vi "GMLAN Diagnostics Engine.vi"(8 "error in (no error)":errorcluster, 11 "State Variables":T1={"TCP Refs"={"Connection List"=refnum, "listener ID"=refnum}, "Stop"=refnum, "Top VI"=refnum, "Parameters"={"Name"="", "PID Lookup"=variant, "DID Lookup"=variant, "Section Properties"={"CAN"={"Database File"=path "", "CAN Interface"=enum."CAN0", "Baud Rate"=0, "Diagnostic Protocol"=enum."GMLAN", "Transport Protocol"=enum."ISO TP - Normal Mode", "Transmit ID"=0, "Receive ID"=0, "Transmit Extension"=0, "Receive Extension"=0, "Receive UUDT ID"=0, "Enable Stream"=TRUE, "VW TP Channel ID"=0}, "DPIDs"=[], "DTC descriptor"={"DTC Byte Length"=2, "Status Byte Length"=1, "Add Data Byte Length"=1, "Byte Order"=enum."Motorola"}, "PIDs"=[], "DIDs"=[], "CPIDs"=[]}, "ChanRefs"={"ToVS.PIDs"={"Name"="", "Write to VS Engine FIFO"=refnum, "Pairs"={"Refs"=[], "Values"=[]}}, "ToVS.DIDs"={"Name"="", "Write to VS Engine FIFO"=refnum, "Pairs"={"Refs"=[], "Values"=[]}}, "ToVS.DTCs"={"Name"="", "Write to VS Engine FIFO"=refnum, "Pairs"={"Refs"=[], "Values"=[]}}, "ToVS.DTCCount"={"Name"="", "Write to VS Engine FIFO"=refnum, "Pairs"={"Refs"=[], "Values"=[]}}, "ToVS.Success"={"Name"="", "Write to VS Engine FIFO"=refnum, "Pairs"={"Refs"=[], "Values"=[]}}, "FromVS.CPIDs"={"Name"="", "Read from VS Engine FIFO"=refnum, "Pairs"={"Refs"=[], "Values"=[]}}, "Cmds"={"Name"="", "Write to VS Engine FIFO"=refnum, "Read from VS Engine FIFO"=refnum, "Pairs"={"Chan Refs"=[], "Prev. Values"=[]}}}, "CPID Lookup"=variant, "DPID Lookup"=variant}, "ADCS Connection"={"Diag CAN Handle"=0, "Transport Protocol"=enum."ISO TP - Normal Mode", "Receive Address Extension"=0, "Transmit Address Extension"=0, "Receive CAN Id"=0, "Transmit CAN Id"=0, "Diag CAN Queue"=refnum, "Log Frames ?"=FALSE, "My TP Address"=0, "Other TP Address"=0, "T1"=0, "T2"=0, "T3"=0, "T4"=0, "Tx SN"=0, "Block Size"=0, "Rx SN"=0, "VW TP Initialized?"=FALSE, "Tx block no"=0, "baud rate"=0, "Interface"="", "Channel Diag CAN Handle"=0, "UDP Connection ID"=refnum, "TCP Connection ID"=refnum, "Target IP Addr"=0, "Source Address"=0, "Target Address"=0, "Send Header NACK?"=FALSE, "DLL Handle"=0, "NAD"=0, "Time Stamp read first"=0.0, "Time Stamp read last"=0.0, "Time Stamp write first"=0.0, "Time Stamp write last"=0.0, "Time Stamp write"=0.0, "Time Stamp read"=0.0}, "XNET References"={"Database"="", "GMLAN DPID Session"="", "Cluster"=""}, "BufferedCmds"=refnum, "XNETEngine (GMLAN)"=refnum} {"Parameters"."ChanRefs"."Cmds"."Pairs"."Chan Refs" format="%.0x"; "Parameters"."ChanRefs"."ToVS.Success"."Pairs"."Refs" format="%.0x"; "Parameters"."ChanRefs"."ToVS.DTCCount"."Pairs"."Refs" format="%.0x"; "Parameters"."ChanRefs"."ToVS.DTCs"."Pairs"."Refs" format="%.0x"; "Parameters"."ChanRefs"."ToVS.PIDs"."Pairs"."Refs" format="%.0x"; "Parameters"."ChanRefs"."ToVS.DIDs"."Pairs"."Refs" format="%.0x"; "Parameters"."Section Properties"."CPIDs"."Signals"."Byte Order" items=["Little Endian", "Big Endian"]; "Parameters"."Section Properties"."CPIDs"."Signals"."Data Type" items=["Signed", "Unsigned", "IEEE Float"]; "Parameters"."Section Properties"."DIDs"."Signals"."Byte Order" items=["Little Endian", "Big Endian"]; "Parameters"."Section Properties"."DIDs"."Signals"."Data Type" items=["Signed", "Unsigned", "IEEE Float"]; "Parameters"."Section Properties"."CAN"."VW TP Channel ID" format="%.0x"; "Parameters"."Section Properties"."CAN"."Receive UUDT ID" format="%.0x"; "Parameters"."Section Properties"."CAN"."Receive Extension" format="%.0x"; "Parameters"."Section Properties"."CAN"."Transmit Extension" format="%.0x"; "Parameters"."Section Properties"."CAN"."Receive ID" format="%.0x"; "Parameters"."Section Properties"."CAN"."Transmit ID" format="%.0x"; "Parameters"."Section Properties"."PIDs"."Signals"."Byte Order" items=["Little Endian", "Big Endian"]; "Parameters"."Section Properties"."PIDs"."Signals"."Data Type" items=["Signed", "Unsigned", "IEEE Float"]}) -> (0 "error out":errorcluster)   [LabVIEW 2013, in "Diagnostics Addon Engine.lvlib"]
uses:
  Diagnostics Addon Engine.lvlib
  State Variables.ctl
  TCP Refs.ctl
  STM/STM Lookup Table Ref.ctl
  Stop FG/Stop Global Ref.ctl
  Main Configuration.ctl
  Section Properties.ctl
  Shared/CAN Configuration.ctl
  Shared/CAN Interface.ctl
  Shared/Diagnostic Protocols.ctl
  Shared/Transport Protocols.ctl
  Shared/DPID Parameters.ctl
  Shared/DPID Periodic Rate.ctl
  <vilib>/Automotive Diagnostic Command Set/Diagnostic Protocols.llb/DTC Descriptor.ctl
  Shared/DIDPID Parameters.ctl
  Shared/DIDPID Signal Parameters.ctl
  VS Data Channels.ctl
  Inline Async API/Controls/Write To VS Engine.ctl
  <vilib>/NI Veristand/Custom Device API/Data Reference.ctl
  Inline Async API/Controls/Read From VS Engine.ctl
  <vilib>/NI Veristand/Custom Device API/Block Data Reference.ctl
  Inline Async API/Controls/ReadWrite Data.ctl
  <vilib>/Automotive Diagnostic Command Set/Diagnostic Transport.llb/Diag Reference.ctl
  <vilib>/Automotive Diagnostic Command Set/Diagnostic Transport.llb/Transport Protocol Selector.ctl
  <vilib>/Automotive Diagnostic Command Set/Diagnostic Transport.llb/Diag CAN Frame Log.ctl
  XNET References.ctl
  <vilib>/NI/AMC/Message Queue.ctl
  <vilib>/NI/AMC/Message.ctl
  <vilib>/NI/Tools/Keyed Array/KeyedArray.ctl
  Stop FG/Stop Global Commands.ctl
  Shared/DTC and Timestamp Cluster.ctl
  GMLAN/_SubVIs/DisableNormalCommunication_Parameter.ctl
  GMLAN/_SubVIs/ReadDataByPacketIdentifier_SubFunctions.ctl
  <vilib>/Automotive Diagnostic Command Set/Diagnostic Transport.llb/Property ID.ctl
  ReadDTCbyDTCNumber Parameters.ctl
  GMLAN/_SubVIs/ReadFailureRecordData_readFailureRecordParameters_failureRecordIdentifier.ctl
  Datatable Lookup Positions.ctl
  PID Data.ctl
  GMLAN/_SubVIs/TesterPresent_Parameter.ctl
  GMLAN/Utilities/GMLAN Service Broadcast.vi
  <vilib>/NI/AMC/Create Single Message.vi
  <vilib>/NI/AMC/Update Message Routing Info.vi
  <vilib>/NI/Tools/Keyed Array/Map String.vi
  <vilib>/NI/AMC/Read Termination Message.vi
  <vilib>/NI/Tools/String/Get Case Matching.vi
  <vilib>/NI/AMC/Globals.vi
  <vilib>/Automotive Diagnostic Command Set/Diagnostic Transport.llb/Apply Success Failure Error.vi
  <vilib>/Automotive Diagnostic Command Set/Diagnostic Transport.llb/Diagnostic Service.vi
  <vilib>/Utility/error.llb/Clear Errors.vi
  Shared/GUID Lookup.vi
  <vilib>/NI/AMC/Send Message.vi
  <vilib>/Automotive Diagnostic Command Set/Diagnostic Transport.llb/Apply Diagnostic Error.vi
  <vilib>/Automotive Diagnostic Command Set/Diagnostic Transport.llb/Diag Globals.vi
  <vilib>/Automotive Diagnostic Command Set/Diagnostic Transport.llb/Diagnostic Service Send.vi
  <vilib>/Automotive Diagnostic Command Set/Diagnostic Transport.llb/Diagnostic Response Recv.vi
  Convert ID to Raw Data.vi
  <vilib>/xnet/xnet.llb/XNET Convert (Frame Raw to Signal).vi
  Stop FG/Stop FG.lvlib
  Shared/Diagnostics Addon Shared.lvlib
  Error Handling API/Error Handling API.lvlib
  <vilib>/NI Veristand/Custom Device Tools/Custom Device Utility Library/Custom Device Utility Library.lvlib
  <vilib>/addons/Automotive Diagnostic Command Set/NI_Automotive Diagnostic Command Set.lvlib
  <vilib>/NI/AMC/AMC.lvlib
  <vilib>/NI/Tools/Keyed Array/Tools_KeyedArray.lvlib
  GMLAN/GMLAN.lvlib
  <vilib>/NI Veristand/Custom Device API/Custom Device API.lvlib
  Inline Async API/Inline Async API.lvlib
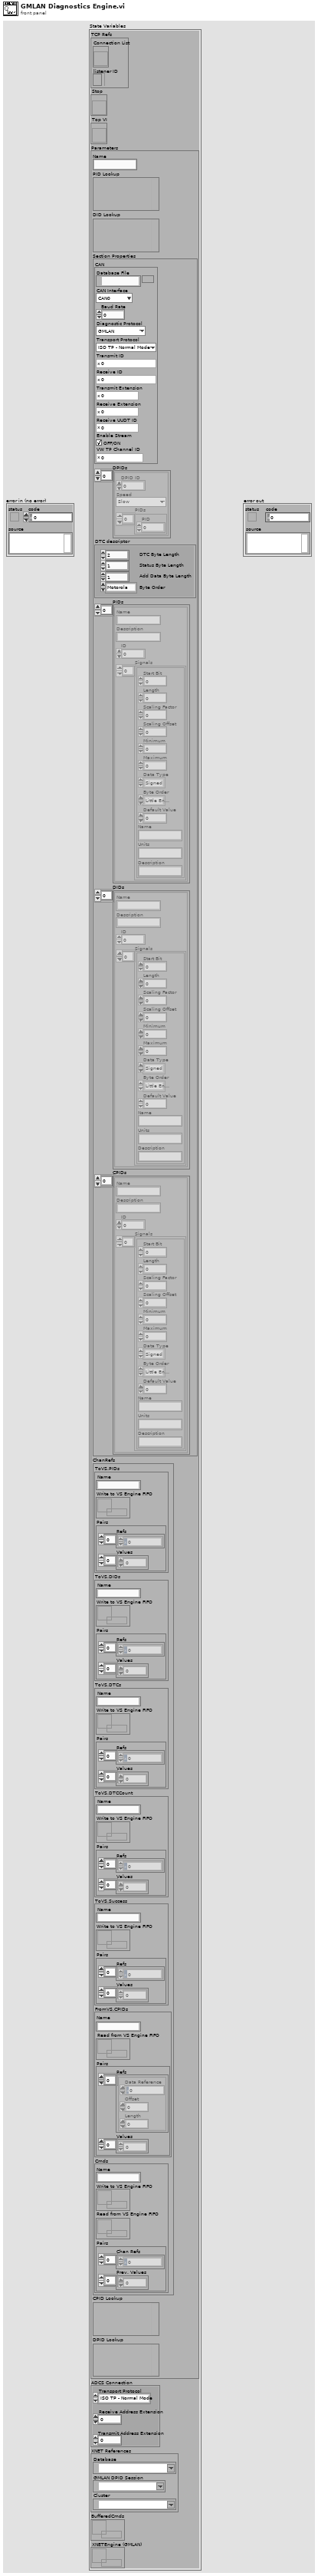
[diagram p1: front panel]
types:
  T1 = typedef "Diagnostics Addon Engine.lvlib/State Variables.ctl" = cluster{"TCP Refs":T2, "Stop":T4, "Top VI":refnum<vi>, "Parameters":T5, "ADCS Connection":T22, "XNET References":T24, "BufferedCmds":T25, "XNETEngine (GMLAN)":T25}
  T2 = typedef "Diagnostics Addon Engine.lvlib/TCP Refs.ctl" = cluster{"Connection List":T3, "listener ID":refnum<k5>}
  T3 = typedef "Diagnostics Addon Engine.lvlib/STM Lookup Table Ref.ctl" = refnum<vi>
  T4 = typedef "Diagnostics Addon Engine.lvlib/Stop FG.lvlib/Stop Global Ref.ctl" = refnum<vi>
  T5 = typedef "Diagnostics Addon Engine.lvlib/Main Configuration.ctl" = cluster{"Name":string, "PID Lookup":variant, "DID Lookup":variant, "Section Properties":T6, "ChanRefs":T16, "CPID Lookup":variant, "DPID Lookup":variant}
  T6 = typedef "Diagnostics Addon Engine.lvlib/Section Properties.ctl" = cluster{"CAN":T7, "DPIDs":T11[], "DTC descriptor":T13, "PIDs":T14[], "DIDs":T14[], "CPIDs":T14[]}
  T7 = typedef "Diagnostics Addon Shared.lvlib/CAN Configuration.ctl" = cluster{"Database File":path, "CAN Interface":T8, "Baud Rate":u32, "Diagnostic Protocol":T9, "Transport Protocol":T10, "Transmit ID":u32, "Receive ID":u32, "Transmit Extension":u8, "Receive Extension":u8, "Receive UUDT ID":u32, "Enable Stream":bool, "VW TP Channel ID":u32}
  T8 = typedef "Diagnostics Addon Shared.lvlib/CAN Interface.ctl" = enum16{"CAN0", "CAN1", "CAN2", "CAN3", "CAN4", "CAN5", "CAN6", "CAN7", "CAN8", "CAN9", "CAN10", "CAN11", "CAN12", "CAN13", "CAN14", "CAN15", "CAN16", "CAN17", "CAN18", "CAN19", "CAN20", "CAN21", "CAN22", "CAN23", "CAN24", "CAN25", "CAN26", "CAN27", "CAN28", "CAN29", "CAN30", "CAN31", "CAN32", "CAN33", "CAN34", "CAN35", "CAN36", "CAN37", "CAN38", "CAN39", "CAN40", "CAN41", "CAN42", "CAN43", "CAN44", "CAN45", "CAN46", "CAN47", "CAN48", "CAN49", "CAN50", "CAN51", "CAN52", "CAN53", "CAN54", "CAN55", "CAN56", "CAN57", "CAN58", "CAN59", "CAN60", "CAN61", "CAN62", "CAN63", "CAN 256 (Virtual)", "CAN 257 (Virtual)"}
  T9 = typedef "Diagnostics Addon Shared.lvlib/Diagnostic Protocols.ctl" = enum16{"GMLAN", "KWP-2000", "UDS"}
  T10 = typedef "Diagnostics Addon Shared.lvlib/Transport Protocols.ctl" = enum16{"ISO TP - Normal Mode", "ISO TP - Mixed Mode", "VW TP 2.0", "Diagnostics on IP"}
  T11 = typedef "Diagnostics Addon Shared.lvlib/DPID Parameters.ctl" = cluster{"DPID ID":u8, "Speed":T12, "PIDs":u16[]}
  T12 = typedef "Diagnostics Addon Shared.lvlib/DPID Periodic Rate.ctl" = enum16{"Slow", "Medium", "Fast"}
  T13 = typedef "DTC Descriptor.ctl" = cluster{"DTC Byte Length":i32, "Status Byte Length":i32, "Add Data Byte Length":i32, "Byte Order":enum16{"Motorola", "Intel"}}
  T14 = typedef "Diagnostics Addon Shared.lvlib/DIDPID Parameters.ctl" = cluster{"Name":string, "Description":string, "ID":u16, "Signals":T15[]}
  T15 = typedef "Diagnostics Addon Shared.lvlib/DIDPID Signal Parameters.ctl" = cluster{"Start Bit":u8, "Length":u8, "Scaling Factor":dbl, "Scaling Offset":dbl, "Minimum":dbl, "Maximum":dbl, "Data Type":u32, "Byte Order":u32, "Default Value":dbl, "Name":string, "Units":string, "Description":string}
  T16 = typedef "Diagnostics Addon Engine.lvlib/VS Data Channels.ctl" = cluster{"ToVS.PIDs":T17, "ToVS.DIDs":T17, "ToVS.DTCs":T17, "ToVS.DTCCount":T17, "ToVS.Success":T17, "FromVS.CPIDs":T19, "Cmds":T21}
  T17 = typedef "Diagnostics Addon Engine.lvlib/Inline Async API.lvlib/Write To VS Engine.ctl" = cluster{"Name":string, "Write to VS Engine FIFO":refnum<k33>, "Pairs":cluster{"Refs":T18[], "Values":dbl[]}}
  T18 = typedef "Custom Device API.lvlib/Data Reference.ctl" = i32
  T19 = typedef "Diagnostics Addon Engine.lvlib/Inline Async API.lvlib/Read From VS Engine.ctl" = cluster{"Name":string, "Read from VS Engine FIFO":refnum<k33>, "Pairs":cluster{"Refs":T20[], "Values":dbl[]}}
  T20 = typedef "Custom Device API.lvlib/Block Data Reference.ctl" = cluster{"Data Reference":T18, "Offset":i32, "Length":i32}
  T21 = typedef "Diagnostics Addon Engine.lvlib/Inline Async API.lvlib/ReadWrite Data.ctl" = cluster{"Name":string, "Write to VS Engine FIFO":refnum<k33>, "Read from VS Engine FIFO":refnum<k33>, "Pairs":cluster{"Chan Refs":T18[], "Prev. Values":dbl[]}}
  T22 = typedef "NI_Automotive Diagnostic Command Set.lvlib/Diag Reference.ctl" = cluster{"Diag CAN Handle":u32, "Transport Protocol":T23, "Receive Address Extension":u8, "Transmit Address Extension":u8, "Receive CAN Id":u32, "Transmit CAN Id":u32, "Diag CAN Queue":refnum<queue>, "Log Frames ?":bool, "My TP Address":u8, "Other TP Address":u8, "T1":u16, "T2":u16, "T3":u16, "T4":u16, "Tx SN":u8, "Block Size":u8, "Rx SN":u8, "VW TP Initialized?":bool, "Tx block no":u8, "baud rate":u32, "Interface":string, "Channel Diag CAN Handle":u32, "UDP Connection ID":refnum<k16>, "TCP Connection ID":refnum<k5>, "Target IP Addr":u32, "Source Address":u16, "Target Address":u16, "Send Header NACK?":bool, "DLL Handle":u32, "NAD":u8, "Time Stamp read first":dbl, "Time Stamp read last":dbl, "Time Stamp write first":dbl, "Time Stamp write last":dbl, "Time Stamp write":dbl, "Time Stamp read":dbl}
  T23 = typedef "NI_Automotive Diagnostic Command Set.lvlib/Transport Protocol Selector.ctl" = enum16{"ISO TP - Normal Mode", "ISO TP - Mixed Mode", "VW TP 2.0", "Diagnostics on IP", "ISO TP LIN"}
  T24 = typedef "Diagnostics Addon Engine.lvlib/XNET References.ctl" = cluster{"Database":refnum<k21>, "GMLAN DPID Session":refnum<k21>, "Cluster":refnum<k21>}
  T25 = typedef "AMC.lvlib/Message Queue.ctl" = refnum<queue>
  T26 = typedef "Diagnostics Addon Shared.lvlib/DTC and Timestamp Cluster.ctl" = cluster{"Timestamp":dbl, "DTC":dbl, "Status":dbl, "Add Data":dbl}
  T27 = typedef "Diagnostics Addon Engine.lvlib/Stop FG.lvlib/Stop Global Commands.ctl" = enum16{"Write", "Read", "Reset"}
  T28 = typedef "GMLAN.lvlib/TesterPresent_Parameter.ctl" = enum8{"SpecificECU", "EntireNetwork"}
  T29 = typedef "GMLAN.lvlib/DisableNormalCommunication_Parameter.ctl" = enum8{"SpecificECU", "EntireNetwork"}
  T30 = typedef "NI_Automotive Diagnostic Command Set.lvlib/Property ID.ctl" = enum16{"Timeout Diag Command", "Timeout FC (Bs)", "Timeout CF (Cr)", "Receive Block Size (BS)", "Wait Time CF (STmin)", "Max Wait Frames (N_WFTmax)", "Wait Frames to Send (N_WAIT)", "Time between Waits (T_W)", "Fill CAN Frames", "Fill Byte", "Invalid Response as Error", "Max RspPending Count", "VWTP Command Timeout", "STmin", "P2min", "Termination"}
  T31 = typedef "GMLAN.lvlib/ReadDataByPacketIdentifier_SubFunctions.ctl" = enum8{"stopSending", "sendOneResponse", "scheduleAtSlowRate", "scheduleAtMediumRate", "scheduleAtFastRate"}
  T32 = typedef "Diagnostics Addon Engine.lvlib/ReadDTCbyDTCNumber Parameters.ctl" = cluster{"DTC":u16, "FailTypeByte":u8}
  T33 = typedef "GMLAN.lvlib/ReadFailureRecordData_readFailureRecordParameters_failureRecordIdentifier.ctl" = cluster{"failureRecordNumber":u8, "DTC ID":u16, "DTCFailureType":u8}
  T34 = enum16{"open", "replace", "create", "open or create", "replace or create", "replace or create with confirmation"}
  T35 = typedef "Diagnostics Addon Engine.lvlib/Datatable Lookup Positions.ctl" = cluster{"Offset":i32, "Length":i32}
  T36 = typedef "Diagnostics Addon Engine.lvlib/PID Data.ctl" = cluster{"ID":u16, "Raw Frame":u8[]}
  T37 = typedef "AMC.lvlib/Message.ctl" = cluster{"name":string, "value":string, "attributes":T38, "receiver host":string, "receiver process":string, "source host":string, "source process":string, "priority message":bool, "acknowledge message":bool}
  T38 = typedef "Tools_KeyedArray.lvlib/KeyedArray.ctl" = cluster{"keys":string[], "values":string[]}
  T39 = typedef "Diagnostics Addon Engine.lvlib/Filtered DPID IDs.ctl" = cluster{"Slow":u8[], "Medium":u8[], "Fast":u8[]}
  T40 = cluster{"Boolean array[0]":bool, "Boolean array[1]":bool, "Boolean array[2]":bool, "Boolean array[3]":bool, "Boolean array[4]":bool, "Boolean array[5]":bool, "Boolean array[6]":bool, "Boolean array[7]":bool}
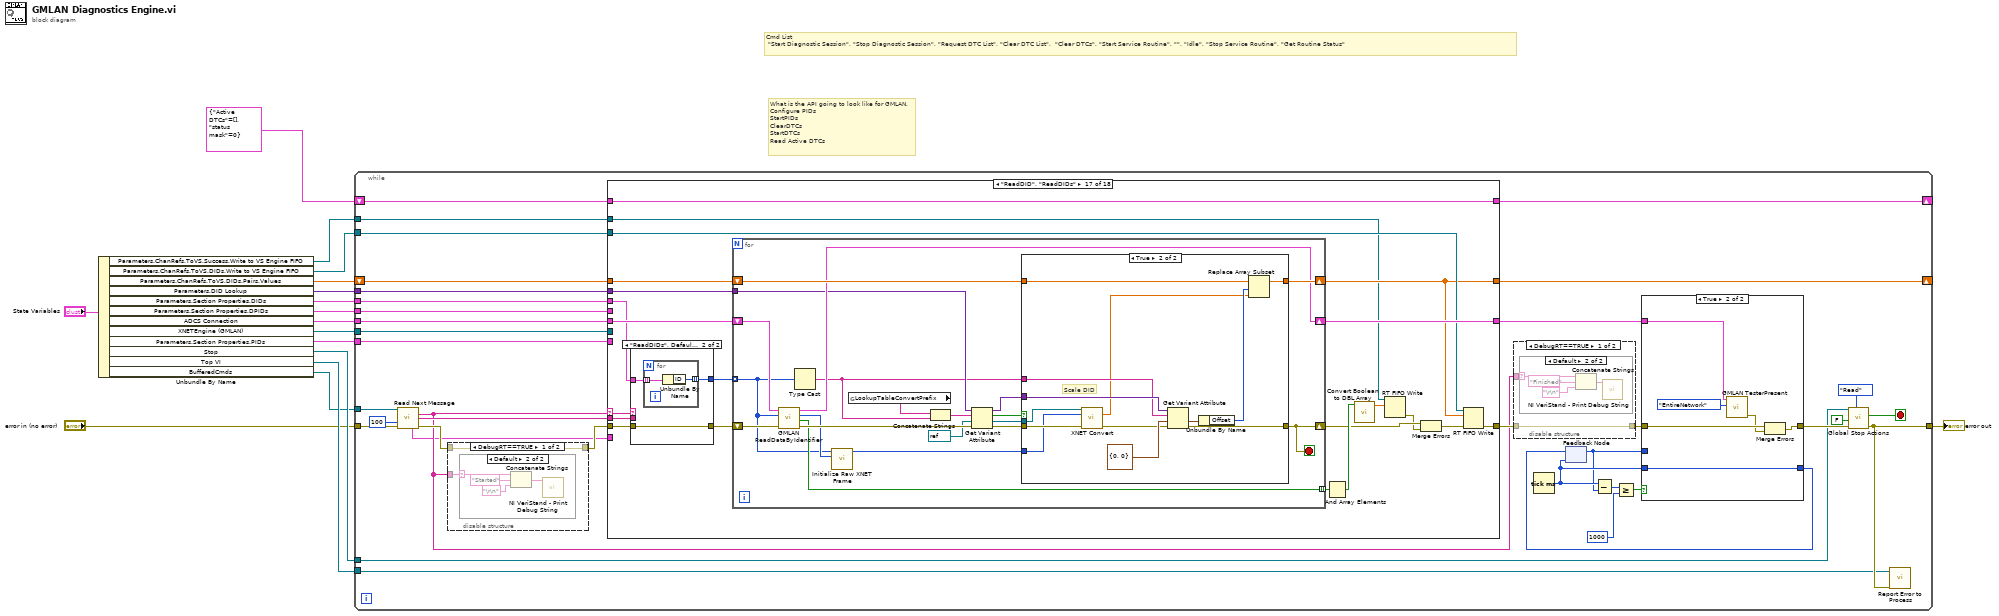
[diagram p0: block diagram]
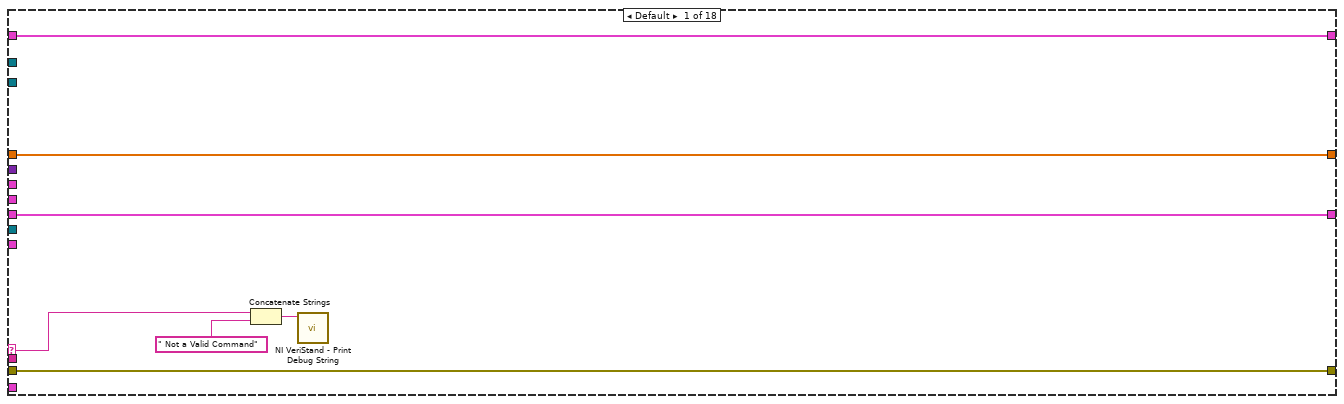
[diagram p7: hidden frame]
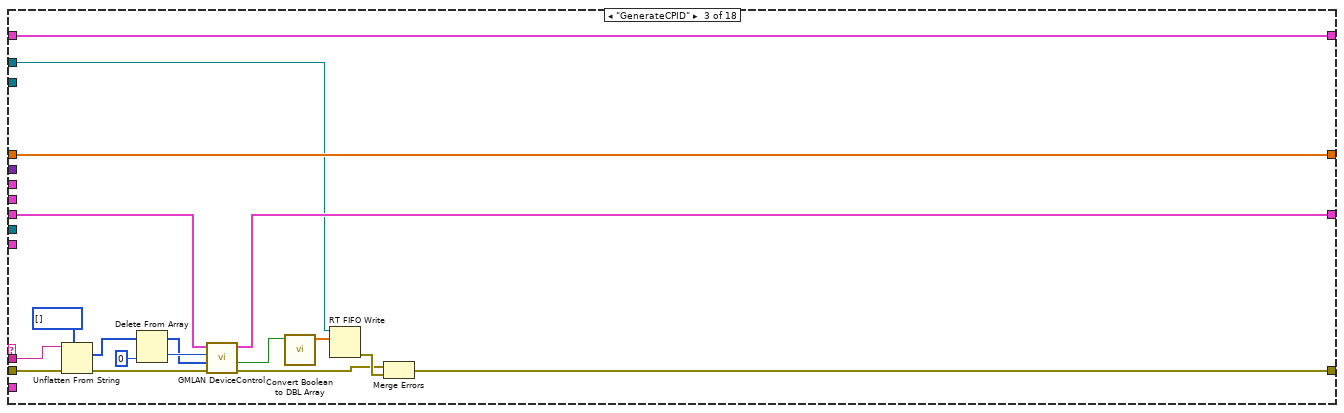
[diagram p9: hidden frame]
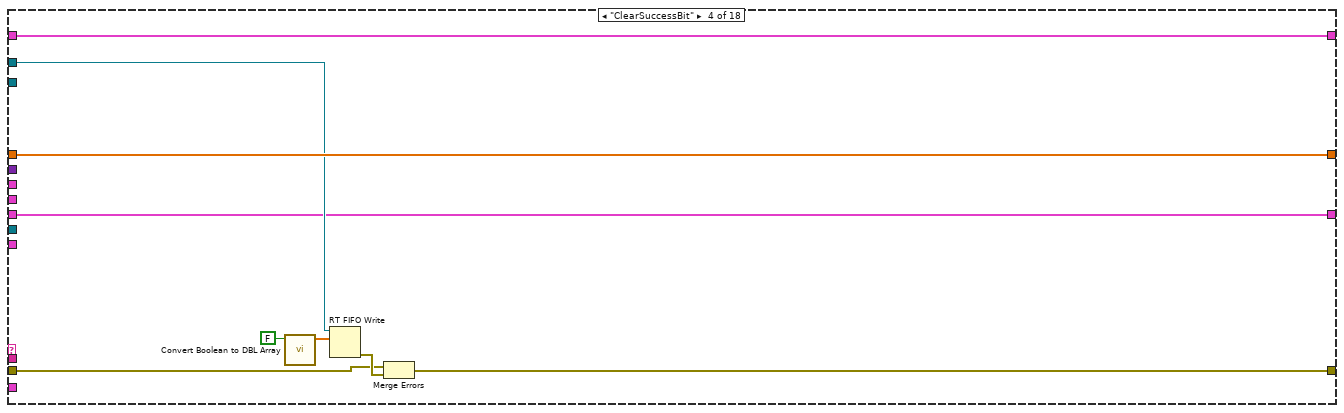
[diagram p10: hidden frame]
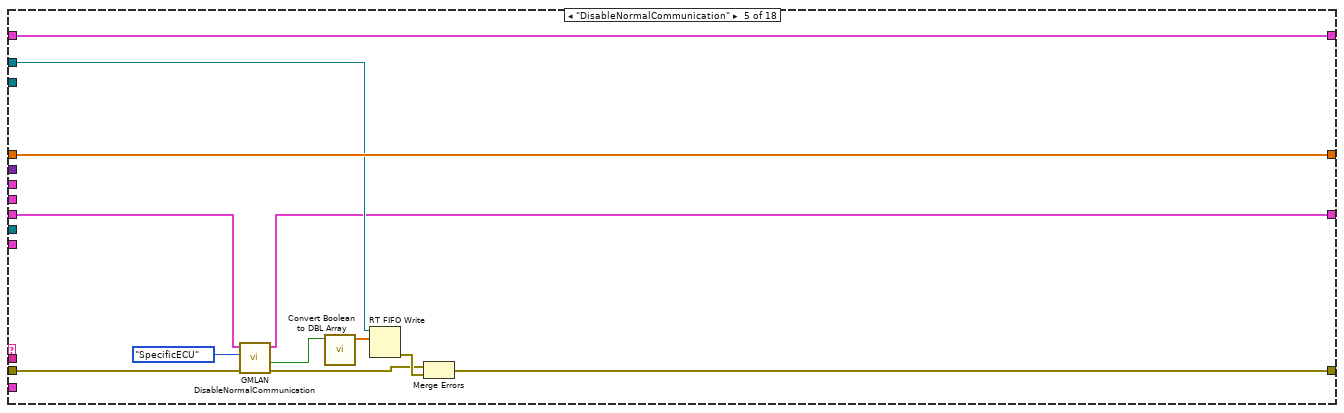
[diagram p11: hidden frame]
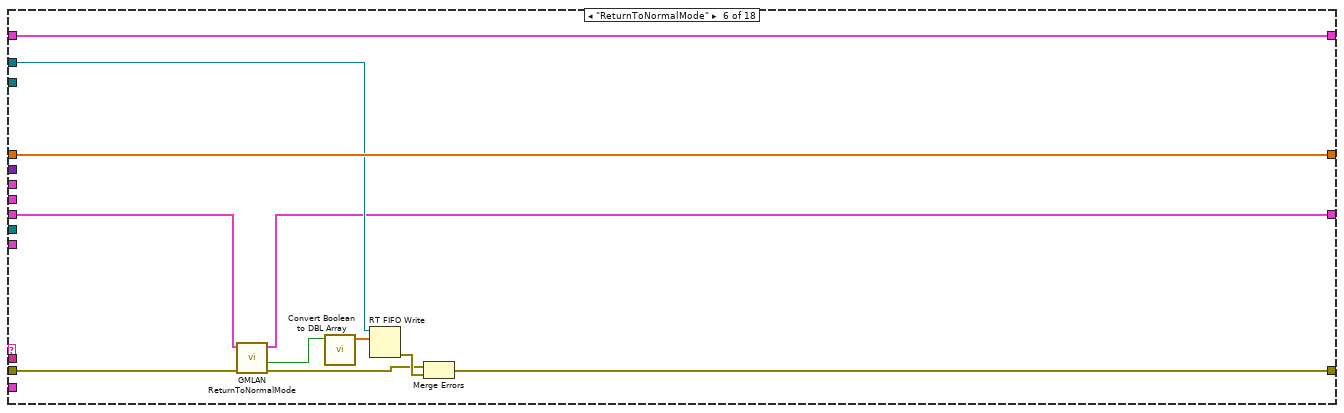
[diagram p12: hidden frame]
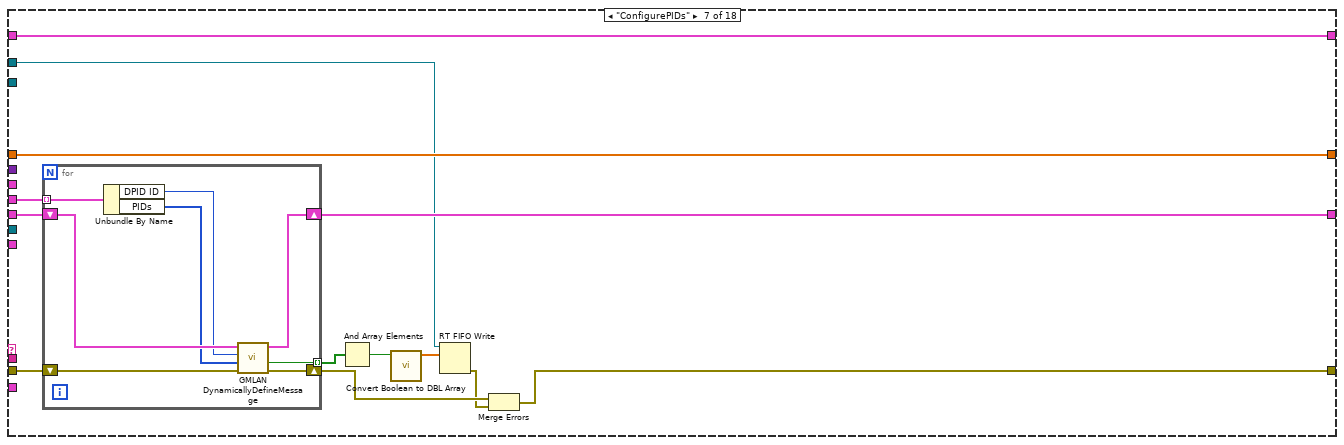
[diagram p13: hidden frame]
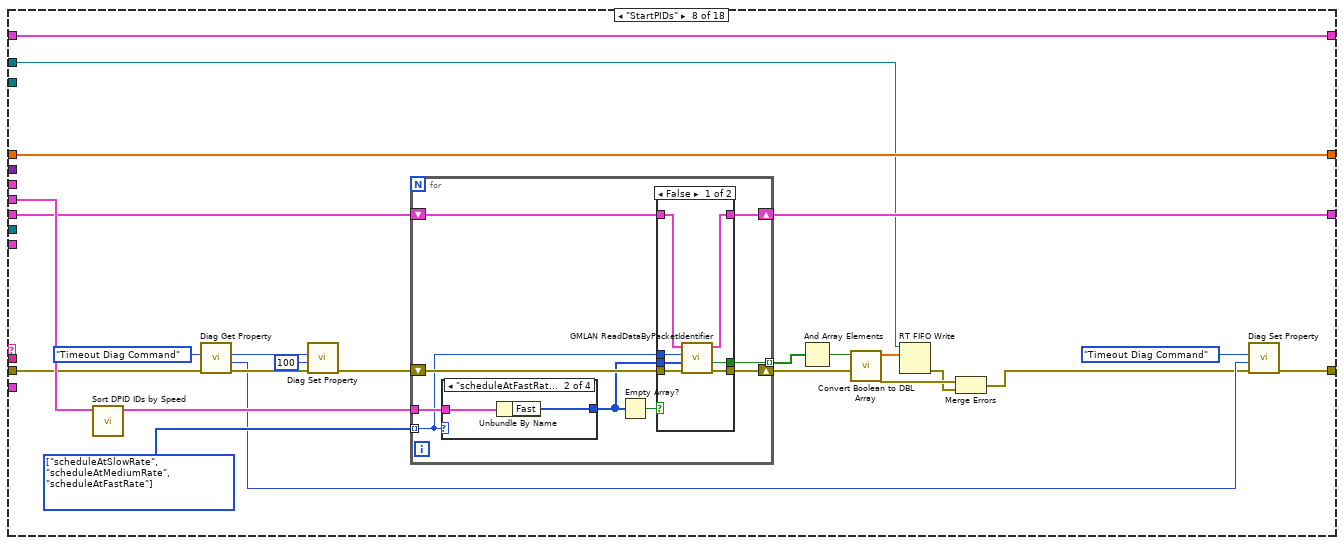
[diagram p14: hidden frame]
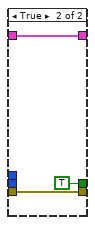
[diagram p15: hidden frame]
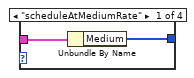
[diagram p16: hidden frame]
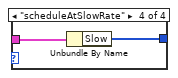
[diagram p18: hidden frame]
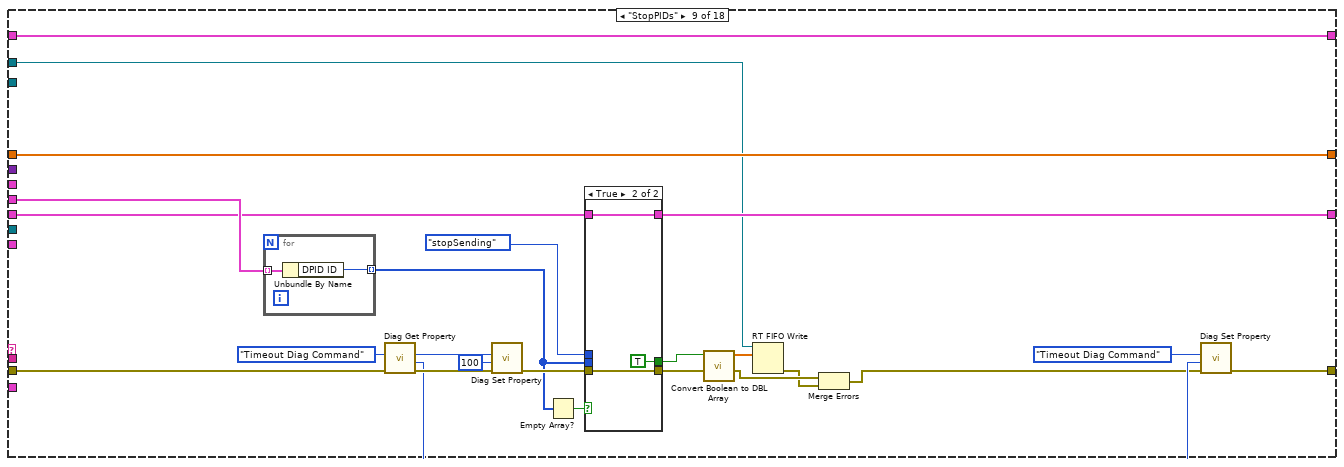
[diagram p19: hidden frame]
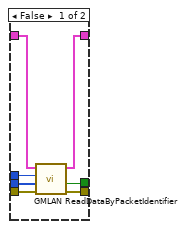
[diagram p20: hidden frame]
diagram:
  # "What is the API going to look like for GMLAN.\nConfigure PIDs\nStartPIDs\nClearDTCs\nStartDTCs\nRead Active DTCs"
  # "Cmd List\n \"Start Diagnostic Session\", \"Stop Diagnostic Session\", \"Request DTC List\", \"Clear DTC List\",  \"Clear DTCs\", \"Start Service Routine\", \"\", \"Idle\", \"Stop Service Routine\", \"Get Routine Status\""
  n1 = Unbundle By Name("State Variables") -> ("Parameters.ChanRefs.ToVS.Success.Write to VS Engine FIFO"=w4:refnum<k33>, "Parameters.ChanRefs.ToVS.DIDs.Write to VS Engine FIFO"=w15:refnum<k33>, "Parameters.ChanRefs.ToVS.DIDs.Pairs.Values"=w11:dbl[], "Parameters.DID Lookup"=w13:variant, "Parameters.Section Properties.DIDs"=w5:T14[], "Parameters.Section Properties.DPIDs"=w8:T11[], "ADCS Connection"=w7:T22, "XNETEngine (GMLAN)"=w16:T25, "Parameters.Section Properties.PIDs"=w2:T14[], "Stop"=w14:T4, "Top VI"=w10:refnum<vi>, "BufferedCmds"=w1:T25)
  n2 = while {
    tunnel: w1 -> [w52]
    tunnel: w7 -> [w46]
    tunnel: w8 -> [w45]
    tunnel: w10 -> [w34]
    tunnel: "error in (no error)" -> [w50]
    tunnel: [w36] -> w9
    shift-right: [w30] -> _
    shift-left: w11 -> [w33]
    tunnel: w13 -> [w32]
    tunnel: w14 -> [w31]
    tunnel: w15 -> [w29]
    tunnel: w16 -> [w28]
    shift-right: [w27] -> _
    shift-left: cluster{"Active DTCs":T26[], "status mask":u8} {"Active DTCs"=[], "status mask"=0} -> [w26]
    tunnel: w5 -> [w20]
    tunnel: w4 -> [w18]
    tunnel: w2 -> [w17]
    stop <- w35 stop-if-true
    n3 = call <vilib>:"Read Next Message.vi"("message queue in"=w52, "timeout (1 ms)"=100 ("timeout (1ms)"), "error in"=w50) -> ("message name"=w21:string, "message value"=w47:string, "message"=w19:T37, "error out"=w23:errorcluster)  [unwired: 5 in, 4 out]
    n4 = disable-structure shown="DebugRT==TRUE" {
      disable-tunnel: w21 -> [w54 _]
      disable-tunnel: [w53 w59] -> w22
      disable-tunnel: w23 -> [w53 w59]
      frame condition #0 {
        n5 = case shown="Default" w54 {
          selector: w54 -> [_ w56]
          frame "" {
          }
          frame Default {
            n6 = Concatenate Strings(w56, "Started" ("string"), "\r\n") -> (w58:string)
            n7 = call <vilib>:"NI VeriStand - Print Debug String.vi"("Message"=w58) -> ()  [unwired: 10 in, 1 out]
          }
        }
      }
      frame condition #1 (active) {
      }
    }
    n8 = case shown="\"ReadDID\", \"ReadDIDs\"" w21 {
      selector: w21 -> [w75 _ _ _ _ _ _ _ _ w251 w268 _ _ _ _ _ w415 w490]
      tunnel: w22 -> [w80 w84 w101 w105 w117 w129 w143 w167 w216 w241 w287 w319 w355 w380 w387 w398 w412 w488]
      tunnel: w47 -> [_ _ w100 _ _ _ _ _ _ _ w286 w318 w354 w379 w386 _ w410 w486]
      tunnel: [w80 w84 w88 w108 w120 w131 w136 w165 w214 w245 w277 w309 w345 w369 w384 w400 w419 w472] -> w24
      tunnel: w46 -> [w81 w85 w94 w106 w116 w127 w148 w177 w224 w257 w285 w317 w353 w377 w388 w401 w423 w493]
      tunnel: w45 -> [_ _ _ _ _ _ w147 w178 w225 _ _ _ _ _ _ _ _ _]
      tunnel: [w81 w85 w93 w106 w115 w126 w146 w174 w223 w256 w275 w307 w343 w367 w388 w401 w422 w492] -> w40
      tunnel: w33 -> [w79 w83 w103 w112 w124 w135 w145 w173 w222 w255 w284 w316 w352 w376 w389 w402 w421 w480]
      tunnel: [w79 w83 w103 w112 w124 w135 w145 w173 w222 w255 w284 w316 w352 w376 w389 w402 w417 w480] -> w30
      tunnel: w32 -> [_ _ _ _ _ _ _ _ _ _ _ _ _ _ _ _ w420 _]
      tunnel: w29 -> [_ _ _ _ _ _ _ _ _ _ _ _ _ _ _ _ w418 _]
      tunnel: w28 -> [_ _ _ _ _ _ _ _ _ w244 _ _ _ _ _ _ _ w471]
      tunnel: [w78 w82 w102 w111 w123 w134 w144 w172 w221 _ w267 w300 w336 w359 w381 w392 w416 w491] -> w27
      tunnel: w26 -> [w78 w82 w102 w111 w123 w134 w144 w172 w221 _ w267 w300 w336 w360 w383 w392 w416 w491]
      tunnel: w19 -> [_ _ _ _ _ _ _ _ _ w239 _ _ _ _ _ w395 _ _]
      tunnel: w20 -> [_ _ _ _ _ _ _ _ _ _ _ _ _ _ _ _ w414 _]
      tunnel: w18 -> [_ _ w86 w107 w119 w130 w140 w160 w208 w248 w273 w305 w341 w365 _ _ w406 w482]
      tunnel: w17 -> [_ _ _ _ _ _ _ _ _ _ _ _ _ _ _ _ _ w479]
      frame Default {
        n9 = Concatenate Strings(w75, " Not a Valid Command" ("string")) -> (w76:string)
        n10 = call <vilib>:"NI VeriStand - Print Debug String.vi"("Message"=w76) -> ()  [unwired: 10 in, 1 out]
      }
      frame "" {
      }
      frame "GenerateCPID" {
        n11 = Unflatten From String(type=u8[] [], binary string=w100, error in (no error)=w101) -> (value=w98:u8[], error out=w92:errorcluster)  [unwired: 2 in, 1 out]
        n12 = Delete From Array(array=w98, index=0) -> (deleted portion=w96:u8, array with subset deleted=w95:u8[])  [unwired: 1 in]
        n13 = call "GMLAN DeviceControl.vi"("error in (no error)"=w92, "CPIDControlBytes"=w95, "CPID ID"=w96, "diag ref in"=w94) -> ("error out"=w89:errorcluster, "success?"=w87:bool, "diag ref out"=w93:T22)  [unwired: 5 in]
        n14 = call "Convert Boolean to DBL Array.vi"("Boolean"=w87) -> ("DBL Array"=w91:dbl[])  [unwired: 10 in]
        n15 = RT FIFO Write(0:w86, 1:w91) -> (11:w90:errorcluster)  [unwired: 3 in, 3 out]
        n16 = Merge Errors(w89, w90) -> (w88:errorcluster)
      }
      frame "ClearSuccessBit" {
        n17 = call "Convert Boolean to DBL Array.vi"("Boolean"=FALSE) -> ("DBL Array"=w110:dbl[])  [unwired: 10 in]
        n18 = RT FIFO Write(0:w107, 1:w110) -> (11:w109:errorcluster)  [unwired: 3 in, 3 out]
        n19 = Merge Errors(w105, w109) -> (w108:errorcluster)
      }
      frame "DisableNormalCommunication" {
        n20 = call "GMLAN DisableNormalCommunication.vi"("error in (no error)"=w117, "Parameter"=DisableNormalCommunication_Parameter."SpecificECU", "diag ref in"=w116) -> ("error out"=w118:errorcluster, "success?"=w114:bool, "diag ref out"=w115:T22)  [unwired: 6 in]
        n21 = call "Convert Boolean to DBL Array.vi"("Boolean"=w114) -> ("DBL Array"=w122:dbl[])  [unwired: 10 in]
        n22 = RT FIFO Write(0:w119, 1:w122) -> (11:w121:errorcluster)  [unwired: 3 in, 3 out]
        n23 = Merge Errors(w118, w121) -> (w120:errorcluster)
      }
      frame "ReturnToNormalMode" {
        n24 = call "GMLAN ReturnToNormalMode.vi"("error in (no error)"=w129, "diag ref in"=w127) -> ("error out"=w128:errorcluster, "success?"=w125:bool, "diag ref out"=w126:T22)  [unwired: 7 in]
        n25 = call "Convert Boolean to DBL Array.vi"("Boolean"=w125) -> ("DBL Array"=w133:dbl[])  [unwired: 10 in]
        n26 = RT FIFO Write(0:w130, 1:w133) -> (11:w132:errorcluster)  [unwired: 3 in, 3 out]
        n27 = Merge Errors(w128, w132) -> (w131:errorcluster)
      }
      frame "ConfigurePIDs" {
        n28 = for {
          shift-right: [w155] -> w146
          shift-left: w148 -> [w156]
          tunnel: w147 -> [w154] mode=indexing
          shift-right: [w150] -> w138
          shift-left: w143 -> [w151]
          tunnel: [w149] -> w142 mode=indexing
          n29 = Unbundle By Name(w154) -> ("DPID ID"=w153:u8, "PIDs"=w152:u16[])
          n30 = call "GMLAN DynamicallyDefineMessage.vi"("error in (no error)"=w151, "PID List"=w152, "DPID ID"=w153, "diag ref in"=w156) -> ("error out"=w150:errorcluster, "success?"=w149:bool, "diag ref out"=w155:T22)  [unwired: 5 in]
        }
        n31 = And Array Elements(Boolean array=w142) -> (logical AND=w141:bool)
        n32 = call "Convert Boolean to DBL Array.vi"("Boolean"=w141) -> ("DBL Array"=w139:dbl[])  [unwired: 10 in]
        n33 = RT FIFO Write(0:w140, 1:w139) -> (11:w137:errorcluster)  [unwired: 3 in, 3 out]
        n34 = Merge Errors(w138, w137) -> (w136:errorcluster)
      }
      frame "StartPIDs" {
        w169 = Property_ID."Timeout Diag Command" ("property ID")
        w176 = T31[] [enum."scheduleAtSlowRate", enum."scheduleAtMediumRate", enum."scheduleAtFastRate"] items=["stopSending", "sendOneResponse", "scheduleAtSlowRate", "scheduleAtMediumRate", "scheduleAtFastRate"]
        n35 = call "Sort DPID IDs by Speed.vi"("DPIDs"=w178) -> ("Filtered DPIDs IDs"=w175:T39)  [unwired: 10 in]
        n36 = call <vilib>:"Diag Get Property.vi"("error in (no error)"=w167, "property ID"=w169) -> ("error out"=w171:errorcluster, "property value"=w164:u32)  [unwired: 7 in, 1 out]
        n37 = call <vilib>:"Diag Set Property.vi"("error in (no error)"=w171, "property value"=u32 100, "property ID"=w169) -> ("error out"=w166:errorcluster)  [unwired: 7 in, 1 out]
        n38 = for {
          tunnel: w175 -> [w183]
          shift-right: [w186] -> w159
          shift-left: w166 -> [w187]
          shift-right: [w184] -> w174
          shift-left: w177 -> [w185]
          tunnel: w176 -> [w180] mode=indexing
          tunnel: [w179] -> w161 mode=indexing
          n39 = case shown="\"scheduleAtFastRate\"" w180 {
            tunnel: w183 -> [w199 w201 _ w203]
            tunnel: [w198 w200 _ w202] -> w182
            frame "scheduleAtMediumRate" {
              n40 = Unbundle By Name(w199) -> ("Medium"=w198:u8[])
            }
            frame "scheduleAtFastRate" {
              n41 = Unbundle By Name(w201) -> ("Fast"=w200:u8[])
            }
            frame Default {
            }
            frame "scheduleAtSlowRate" {
              n42 = Unbundle By Name(w203) -> ("Slow"=w202:u8[])
            }
          }
          n43 = Empty Array?(array=w182) -> (empty?=w181:bool)
          n44 = case shown="False" w181 {
            tunnel: w187 -> [w194 w196]
            tunnel: [w193 w196] -> w186
            tunnel: w185 -> [w192 w197]
            tunnel: [w191 w197] -> w184
            tunnel: w180 -> [w188 _]
            tunnel: w182 -> [w190 _]
            tunnel: [w189 TRUE ("success?")] -> w179
            frame False {
              n45 = call "GMLAN ReadDataByPacketIdentifier.vi"("error in (no error)"=w194, "DPIDs"=w190, "Sub Function"=w188, "diag ref in"=w192) -> ("error out"=w193:errorcluster, "success?"=w189:bool, "diag ref out"=w191:T22)  [unwired: 4 in, 1 out]
            }
            frame True {
            }
          }
        }
        n46 = And Array Elements(Boolean array=w161) -> (logical AND=w163:bool)
        n47 = call "Convert Boolean to DBL Array.vi"("Boolean"=w163) -> ("DBL Array"=w162:dbl[])  [unwired: 10 in]
        n48 = RT FIFO Write(0:w160, 1:w162) -> (11:w158:errorcluster)  [unwired: 3 in, 3 out]
        n49 = Merge Errors(w159, w158) -> (w157:errorcluster)
        n50 = call <vilib>:"Diag Set Property.vi"("error in (no error)"=w157, "property value"=w164, "property ID"=Property_ID."Timeout Diag Command") -> ("error out"=w165:errorcluster)  [unwired: 7 in, 1 out]
      }
      frame "StopPIDs" {
        w218 = Property_ID."Timeout Diag Command" ("property ID")
        n51 = for {
          tunnel: w225 -> [w237] mode=indexing
          tunnel: [w236] -> w211 mode=indexing
          n52 = Unbundle By Name(w237) -> ("DPID ID"=w236:u8)
        }
        n53 = call <vilib>:"Diag Get Property.vi"("error in (no error)"=w216, "property ID"=w218) -> ("error out"=w220:errorcluster, "property value"=w213:u32)  [unwired: 7 in, 1 out]
        n54 = call <vilib>:"Diag Set Property.vi"("error in (no error)"=w220, "property value"=u32 100, "property ID"=w218) -> ("error out"=w215:errorcluster)  [unwired: 7 in, 1 out]
        n55 = Empty Array?(array=w211) -> (empty?=w212:bool)
        n56 = case shown="True" w212 {
          tunnel: w215 -> [w232 w234]
          tunnel: [w231 w234] -> w207
          tunnel: w224 -> [w230 w235]
          tunnel: [w229 w235] -> w223
          tunnel: ReadDataByPacketIdentifier_SubFunctions."stopSending" ("Sub Function") -> [w228 _]
          tunnel: w211 -> [w227 _]
          tunnel: [w226 TRUE ("success?")] -> w209
          frame False {
            n57 = call "GMLAN ReadDataByPacketIdentifier.vi"("error in (no error)"=w232, "DPIDs"=w227, "Sub Function"=w228, "diag ref in"=w230) -> ("error out"=w231:errorcluster, "success?"=w226:bool, "diag ref out"=w229:T22)  [unwired: 4 in, 1 out]
          }
          frame True {
          }
        }
        n58 = call "Convert Boolean to DBL Array.vi"("Boolean"=w209) -> ("DBL Array"=w210:dbl[])  [unwired: 10 in]
        n59 = RT FIFO Write(0:w208, 1:w210) -> (11:w206:errorcluster)  [unwired: 3 in, 3 out]
        n60 = Merge Errors(w207, w206) -> (w205:errorcluster)
        n61 = call <vilib>:"Diag Set Property.vi"("error in (no error)"=w205, "property value"=w213, "property ID"=Property_ID."Timeout Diag Command") -> ("error out"=w214:errorcluster)  [unwired: 7 in, 1 out]
      }
      frame "ClearDTCs" {
        n62 = Unbundle By Name(w239) -> ("attributes"=w238:T38)
        n63 = global read "GUID Lookup.vi" "ResponseQKey"() -> (w240:string)
        n64 = call <vilib>:"Index.vi"("key"=w240, "array in"=w238) -> ("value"=w243:string)  [unwired: 3 in, 2 out]
        n65 = Empty String/Path?(string/path=w243) -> (empty?=w242:bool)
        n66 = call <vilib>:"Send Local Message.vi"("message queue in"=w244, "message name"="ClearDTCs" ("Message Name"), "error in"=w241) -> ("error out"=w254:errorcluster)  [unwired: 10 in, 2 out]
        n67 = call "GMLAN ClearDiagnosticInformation.vi"("error in (no error)"=w254, "diag ref in"=w257) -> ("error out"=w252:errorcluster, "success?"=w249:bool, "diag ref out"=w256:T22)  [unwired: 7 in]
        n68 = case shown="False" w242 {
          tunnel: w252 -> [w262 w263]
          tunnel: [w261 w263] -> w247
          tunnel: w243 -> [w259 _]
          tunnel: w251 -> [w258 _]
          frame False {
            n69 = call <vilib>:"Send Local Message.vi"("receiver process (\"\" - local)"=w259, "message name"=w258, "message value"="Cleared" ("Message Value"), "error in"=w262) -> ("error out"=w261:errorcluster)  [unwired: 9 in, 2 out]
          }
          frame True {
          }
        }
        n70 = call "Convert Boolean to DBL Array.vi"("Boolean"=w249) -> ("DBL Array"=w250:dbl[])  [unwired: 10 in]
        n71 = RT FIFO Write(0:w248, 1:w250) -> (11:w246:errorcluster)  [unwired: 3 in, 3 out]
        n72 = Merge Errors(w247, w246) -> (w245:errorcluster)
      }
      frame "DTCCountChanged", "StartDTCs" {
        w281 = Property_ID."Timeout Diag Command" ("property ID")
        n73 = case shown="Default" w268 {
          tunnel: w287 -> [w290 w295]
          tunnel: w286 -> [_ w294]
          tunnel: [w288 w292] -> w266
          tunnel: [w290 w291] -> w279
          tunnel: w267 -> [w289 _]
          frame "DTCCountChanged" {
            n74 = Unbundle By Name(w289) -> ("status mask"=w288:u8)
          }
          frame Default {
            n75 = Unflatten From String(type=u8 0 ("status mask"), binary string=w294, error in (no error)=w295) -> (value=w292:u8, error out=w291:errorcluster)  [unwired: 2 in, 1 out]
          }
        }
        n76 = Number To Boolean Array(number=w266) -> (Boolean array=w265:bool[])
        n77 = Array To Cluster(array=w265) -> (cluster=w264:T40)
        n78 = call <vilib>:"Diag Get Property.vi"("error in (no error)"=w279, "property ID"=w281) -> ("error out"=w283:errorcluster, "property value"=w276:u32)  [unwired: 7 in, 1 out]
        n79 = call <vilib>:"Diag Set Property.vi"("error in (no error)"=w283, "property value"=u32 100, "property ID"=w281) -> ("error out"=w278:errorcluster)  [unwired: 7 in, 1 out]
        n80 = call "ReadDiagnosticInformation_ByStatus.vi"("error in (no error)"=w278, "status mask"=w264, "diag ref in"=w285) -> ("error out"=w271:errorcluster, "success?"=w272:bool, "diag ref out"=w275:T22)  [unwired: 5 in, 1 out]
        n81 = call "Convert Boolean to DBL Array.vi"("Boolean"=w272) -> ("DBL Array"=w274:dbl[])  [unwired: 10 in]
        n82 = RT FIFO Write(0:w273, 1:w274) -> (11:w270:errorcluster)  [unwired: 3 in, 3 out]
        n83 = Merge Errors(w271, w270) -> (w269:errorcluster)
        n84 = call <vilib>:"Diag Set Property.vi"("error in (no error)"=w269, "property value"=w276, "property ID"=Property_ID."Timeout Diag Command") -> ("error out"=w277:errorcluster)  [unwired: 7 in, 1 out]
      }
      frame "ReadDTCByDTCNumber" {
        w313 = Property_ID."Timeout Diag Command" ("property ID")
        n85 = Unflatten From String(type=T32 {"DTC"=0, "FailTypeByte"=0}, binary string=w318, error in (no error)=w319) -> (value=w298:T32, error out=w311:errorcluster)  [unwired: 2 in, 1 out]
        n86 = call <vilib>:"Diag Get Property.vi"("error in (no error)"=w311, "property ID"=w313) -> ("error out"=w315:errorcluster, "property value"=w308:u32)  [unwired: 7 in, 1 out]
        n87 = Unbundle By Name(w298) -> ("DTC"=w297:u16, "FailTypeByte"=w296:u8)
        n88 = call <vilib>:"Diag Set Property.vi"("error in (no error)"=w315, "property value"=u32 100, "property ID"=w313) -> ("error out"=w310:errorcluster)  [unwired: 7 in, 1 out]
        n89 = call "ReadDiagnosticInformation_readStatusOfDTCByDTCNumber.vi"("error in (no error)"=w310, "FailTypeByte"=w296, "DTC"=w297, "diag ref in"=w317) -> ("error out"=w303:errorcluster, "success?"=w304:bool, "diag ref out"=w307:T22)  [unwired: 4 in, 1 out]
        n90 = call "Convert Boolean to DBL Array.vi"("Boolean"=w304) -> ("DBL Array"=w306:dbl[])  [unwired: 10 in]
        n91 = RT FIFO Write(0:w305, 1:w306) -> (11:w302:errorcluster)  [unwired: 3 in, 3 out]
        n92 = Merge Errors(w303, w302) -> (w301:errorcluster)
        n93 = call <vilib>:"Diag Set Property.vi"("error in (no error)"=w301, "property value"=w308, "property ID"=Property_ID."Timeout Diag Command") -> ("error out"=w309:errorcluster)  [unwired: 7 in, 1 out]
      }
      frame "ReadFailureRecordParameters" {
        w349 = Property_ID."Timeout Diag Command" ("property ID")
        n94 = Unflatten From String(type=T33 {"failureRecordNumber"=0, "DTC ID"=0, "DTCFailureType"=0} ("failureRecordIdentifier"), binary string=w354, error in (no error)=w355) -> (value=w320:T33, error out=w347:errorcluster)  [unwired: 2 in, 1 out]
        n95 = Unbundle By Name(w320) -> ("DTC ID"=w326:u16, "DTCFailureType"=w325:u8, "failureRecordNumber"=w324:u8)
        n96 = call <vilib>:"Diag Get Property.vi"("error in (no error)"=w347, "property ID"=w349) -> ("error out"=w351:errorcluster, "property value"=w344:u32)  [unwired: 7 in, 1 out]
        n97 = call <vilib>:"Diag Set Property.vi"("error in (no error)"=w351, "property value"=u32 1000, "property ID"=w349) -> ("error out"=w346:errorcluster)  [unwired: 7 in, 1 out]
        n98 = Format Into String(format string="%x, %x, %x" ("initial string"), w326, w325, w324) -> (resulting string=w323:string)  [unwired: 2 in, 1 out]
        n99 = call <vilib>:"NI VeriStand - Print Debug String.vi"("Message"=w323) -> ()  [unwired: 10 in, 1 out]
        n100 = call "ReadFailureRecordData_readFailureRecordParameters.vi"("error in (no error)"=w346, "failureRecordIdentifier"=w320, "diag ref in"=w353) -> ("error out"=w339:errorcluster, "success?"=w340:bool, "data out"=w331:u8[], "diag ref out"=w343:T22)  [unwired: 5 in]
        n101 = Open/Create/Replace File(file path (use dialog)=path "C:/ReadFailureRecordParameters.txt", operation (0:open)=T34."replace or create") -> (refnum out=w329:refnum<file>, error out=w333:errorcluster)  [unwired: 4 in, 1 out]
        n102 = Array To Spreadsheet String(array=w331, 3:"%x" ("format string")) -> (spreadsheet string=w327:string)  [unwired: 1 in]
        n103 = Write to Text File(file (use dialog)=w329, text=w327, error in=w333) -> (refnum out=w328:refnum<file>, error out=w332:errorcluster)  [unwired: 1 in, 1 out]
        n104 = call "Convert Boolean to DBL Array.vi"("Boolean"=w340) -> ("DBL Array"=w342:dbl[])  [unwired: 10 in]
        n105 = RT FIFO Write(0:w341, 1:w342) -> (11:w338:errorcluster)  [unwired: 3 in, 3 out]
        n106 = Close File(refnum=w328, error in=w332) -> ()  [unwired: 2 out]
        n107 = Merge Errors(w339, w338) -> (w337:errorcluster)
        n108 = call <vilib>:"Diag Set Property.vi"("error in (no error)"=w337, "property value"=w344, "property ID"=Property_ID."Timeout Diag Command") -> ("error out"=w345:errorcluster)  [unwired: 7 in, 1 out]
      }
      frame "DisableChangeDTCCount", "EnableChangeDTCCount" {
        w373 = Property_ID."Timeout Diag Command" ("property ID")
        n109 = Unflatten From String(type=u8 0 ("status mask"), binary string=w379, error in (no error)=w380) -> (value=w357:u8, error out=w371:errorcluster)  [unwired: 2 in, 1 out]
        n110 = Bundle By Name(cluster=w360, "status mask"=w357) -> (w359:cluster{"Active DTCs":T26[], "status mask":u8})
        n111 = Number To Boolean Array(number=w357) -> (Boolean array=w358:bool[])
        n112 = Array To Cluster(array=w358) -> (cluster=w356:T40)
        n113 = call <vilib>:"Diag Get Property.vi"("error in (no error)"=w371, "property ID"=w373) -> ("error out"=w375:errorcluster, "property value"=w368:u32)  [unwired: 7 in, 1 out]
        n114 = call <vilib>:"Diag Set Property.vi"("error in (no error)"=w375, "property value"=u32 100, "property ID"=w373) -> ("error out"=w370:errorcluster)  [unwired: 7 in, 1 out]
        n115 = call "ReadDiagnosticInformation_sendOnChangeDTCCount.vi"("error in (no error)"=w370, "status mask"=w356, "diag ref in"=w377) -> ("error out"=w363:errorcluster, "success?"=w364:bool, "diag ref out"=w367:T22)  [unwired: 5 in, 1 out]
        n116 = call "Convert Boolean to DBL Array.vi"("Boolean"=w364) -> ("DBL Array"=w366:dbl[])  [unwired: 10 in]
        n117 = RT FIFO Write(0:w365, 1:w366) -> (11:w362:errorcluster)  [unwired: 3 in, 3 out]
        n118 = Merge Errors(w363, w362) -> (w361:errorcluster)
        n119 = call <vilib>:"Diag Set Property.vi"("error in (no error)"=w361, "property value"=w368, "property ID"=Property_ID."Timeout Diag Command") -> ("error out"=w369:errorcluster)  [unwired: 7 in, 1 out]
      }
      frame "UpdateDTCReport" {
        n120 = Unflatten From String(type=T26[] [] ("Active DTCs"), binary string=w386, error in (no error)=w387) -> (value=w382:T26[], error out=w384:errorcluster)  [unwired: 2 in, 1 out]
        n121 = Bundle By Name(cluster=w383, "Active DTCs"=w382) -> (w381:cluster{"Active DTCs":T26[], "status mask":u8})
      }
      frame "ReadActiveDTCs" {
        n122 = Unbundle By Name(w395) -> ("attributes"=w390:T38)
        n123 = global read "GUID Lookup.vi" "ResponseQKey"() -> (w393:string)
        n124 = Unbundle By Name(w392) -> ("Active DTCs"=w391:T26[])
        n125 = Flatten To String(anything=w391, error in (no error)=w398) -> (data string=w396:string, error out=w397:errorcluster)  [unwired: 2 in, 1 out]
        n126 = call <vilib>:"Index.vi"("key"=w393, "array in"=w390) -> ("value"=w394:string)  [unwired: 3 in, 2 out]
        n127 = call <vilib>:"Send Local Message.vi"("receiver process (\"\" - local)"=w394, "message name"="ActiveDTCs" ("Message Name"), "message value"=w396, "error in"=w397) -> ("error out"=w400:errorcluster)  [unwired: 9 in, 2 out]
      }
      frame "ReadDID", "ReadDIDs" {
        n128 = case shown="\"ReadDIDs\", Default" w415 {
          tunnel: w414 -> [_ w432]
          tunnel: [w424 w431] -> w413
          tunnel: w412 -> [w429 w430]
          tunnel: [w428 w430] -> w411
          tunnel: w410 -> [w426 _]
          frame "ReadDID" {
            n129 = Unflatten From String(type=u16 0 ("ID"), binary string=w426, error in (no error)=w429) -> (value=w425:u16, error out=w428:errorcluster)  [unwired: 2 in, 1 out]
            n130 = Build Array(w425) -> (w424:u16[])
          }
          frame "ReadDIDs", Default {
            n131 = for {
              tunnel: w432 -> [w434] mode=indexing
              tunnel: [w433] -> w431 mode=indexing
              n132 = Unbundle By Name(w434) -> ("ID"=w433:u16)
            }
          }
        }
        n133 = for {
          shift-right: [w437] -> w405
          shift-left: w411 -> [w454]
          shift-right: [w450] -> w422
          shift-left: w423 -> [w453]
          shift-right: [w451] -> w417
          shift-left: w421 -> [w452]
          tunnel: w420 -> [w448]
          tunnel: w413 -> [w435] mode=indexing
          tunnel: [w438] -> w407 mode=indexing
          stop <- w437 stop-if-true
          n134 = call "GMLAN ReadDataByIdentifier.vi"("error in (no error)"=w454, "Data ID (DID)"=w435, "diag ref in"=w453) -> ("error out"=w447:errorcluster, "success?"=w438:bool, "data out"=w436:u8[], "diag ref out"=w450:T22)  [unwired: 5 in]
          n135 = Type Cast(x=w435) -> (*(type *) &x=w440:string)  [unwired: 1 in]
          n136 = call "Initialize Raw XNET Frame.vi"("Data"=w436, "identifier"=w435) -> ("Raw Frame"=w442:u8[])  [unwired: 9 in]
          n137 = global read "GUID Lookup.vi" "LookupTableConvertPrefix"() -> (w449:string)
          n138 = Concatenate Strings(w449, w440) -> (w445:string)
          n139 = Get Variant Attribute(Variant=w448, name=w445, default value (empty Variant)=refnum<k21> refnum ("DID Conversion"), error in=w447) -> (duplicate Variant=w441:variant, found=w439:bool, value=w443:refnum<k21>, error out=w446:errorcluster)
          n140 = case shown="True" w439 {
            tunnel: w452 -> [w456 w468]
            tunnel: [w456 w467] -> w451
            tunnel: [w455 w465] -> w437
            tunnel: w446 -> [w455 w464]
            tunnel: w443 -> [_ w463]
            tunnel: w442 -> [_ w462]
            tunnel: w441 -> [_ w461]
            tunnel: w440 -> [_ w460]
            frame False {
              n141 = disable-structure shown="DebugRT==TRUE" {
                frame condition #0 {
                  # "DLE NOTE - ERROR!!"
                  n142 = call <vilib>:"NI VeriStand - Print Debug String.vi"("Message"="Debug Error-DID Scaling Note Found!!" ("Debug String")) -> ()  [unwired: 10 in, 1 out]
                }
                frame condition #1 (active) {
                }
              }
            }
            frame True {
              # "Scale DID"
              n143 = call-poly <vilib>:"XNET Convert.vi"("session in"=w463, "frame data"=w462, "error in (no error)"=w464) -> ("signal data"=w458:dbl[], "error out"=w466:errorcluster)  [unwired: 10 in, 1 out]
              n144 = Get Variant Attribute(Variant=w461, name=w460, default value (empty Variant)=T35 {"Offset"=0, "Length"=0} ("cluster"), error in=w466) -> (value=w470:T35, error out=w465:errorcluster)  [unwired: 2 out]
              n145 = Unbundle By Name(w470) -> ("Offset"=w459:i32)
              n146 = Replace Array Subset(array=w468, new element=w458, index=w459) -> (w467:dbl[])
            }
          }
        }
        n147 = And Array Elements(Boolean array=w407) -> (logical AND=w409:bool)
        n148 = call "Convert Boolean to DBL Array.vi"("Boolean"=w409) -> ("DBL Array"=w408:dbl[])  [unwired: 10 in]
        n149 = RT FIFO Write(0:w406, 1:w408) -> (11:w403:errorcluster)  [unwired: 3 in, 3 out]
        n150 = Merge Errors(w405, w403) -> (w404:errorcluster)
        n151 = RT FIFO Write(0:w418, 1:w417, 3:w404) -> (11:w419:errorcluster)  [unwired: 2 in, 3 out]
      }
      frame "ReadPIDOnDemand", "ReadPIDsOnDemand" {
        n152 = case shown="\"ReadPIDsOnDemand\", Default" w490 {
          tunnel: w479 -> [_ w502]
          tunnel: [w494 w501] -> w489
          tunnel: w488 -> [w499 w500]
          tunnel: [w498 w500] -> w487
          tunnel: w486 -> [w496 _]
          frame "ReadPIDOnDemand" {
            n153 = Unflatten From String(type=u16 0 ("ID"), binary string=w496, error in (no error)=w499) -> (value=w495:u16, error out=w498:errorcluster)  [unwired: 2 in, 1 out]
            n154 = Build Array(w495) -> (w494:u16[])
          }
          frame "ReadPIDsOnDemand", Default {
            n155 = for {
              tunnel: w502 -> [w504] mode=indexing
              tunnel: [w503] -> w501 mode=indexing
              n156 = Unbundle By Name(w504) -> ("ID"=w503:u16)
            }
          }
        }
        n157 = for {
          shift-right: [w510] -> w476
          shift-left: w487 -> [w514]
          shift-right: [w512] -> w492
          shift-left: w493 -> [w513]
          tunnel: w489 -> [w509] mode=indexing
          tunnel: [w511] -> w483 mode=indexing
          tunnel: [w507] -> w474 mode=indexing
          stop <- w510 stop-if-true
          n158 = call "GMLAN ReadDataByParameterIdentifier.vi"("error in (no error)"=w514, "Parameter ID (PID)"=w509, "diag ref in"=w513) -> ("error out"=w510:errorcluster, "success?"=w511:bool, "data out"=w508:u8[], "diag ref out"=w512:T22)  [unwired: 5 in]
          n159 = call "Initialize Raw XNET Frame.vi"("Data"=w508, "identifier"=w509) -> ("Raw Frame"=w505:u8[])  [unwired: 9 in]
          n160 = Bundle By Name(cluster=T36 {"ID"=0, "Raw Frame"=[]}, "Raw Frame"=w505, "ID"=w509) -> (w507:T36)
        }
        n161 = Flatten To String(anything=w474, error in (no error)=w476) -> (data string=w473:string, error out=w475:errorcluster)  [unwired: 2 in, 1 out]
        n162 = call <vilib>:"Send Local Message.vi"("message queue in"=w471, "message name"="UpdatePIDsOnDemand" ("Message Name"), "message value"=w473, "error in"=w475) -> ("error out"=w477:errorcluster)  [unwired: 9 in, 2 out]
        n163 = And Array Elements(Boolean array=w483) -> (logical AND=w485:bool)
        n164 = call "Convert Boolean to DBL Array.vi"("Boolean"=w485) -> ("DBL Array"=w484:dbl[])  [unwired: 10 in]
        n165 = RT FIFO Write(0:w482, 1:w484) -> (11:w481:errorcluster)  [unwired: 3 in, 3 out]
        n166 = Merge Errors(w477, w481) -> (w472:errorcluster)
      }
    }
    n167 = disable-structure shown="DebugRT==TRUE" {
      disable-tunnel: w21 -> [w60 _]
      disable-tunnel: [w61 w66] -> w25
      disable-tunnel: w24 -> [w61 w66]
      frame condition #0 {
        n168 = case shown="Default" w60 {
          selector: w60 -> [_ w63]
          frame "" {
          }
          frame Default {
            n169 = Concatenate Strings(w63, "Finished" ("string"), "\r\n") -> (w65:string)
            n170 = call <vilib>:"NI VeriStand - Print Debug String.vi"("Message"=w65) -> ()  [unwired: 10 in, 1 out]
          }
        }
      }
      frame condition #1 (active) {
      }
    }
    n171 = Tick Count (ms)() -> (millisecond timer value=w42:u32)
    n172 = feedback #1(w42) -> (w41:u32)
    n173 = Subtract(x=w42, y=w41) -> (x-y=w49:u32)
    n174 = Greater Or Equal?(x=w49, y=u32 1000) -> (x >= y?=w44:bool)
    n175 = case shown="True" w44 {
      tunnel: w25 -> [w67 w72]
      tunnel: [w68 w74] -> w43
      tunnel: w41 -> [w68 _]
      tunnel: w42 -> [_ w74]
      tunnel: w40 -> [_ w73]
      tunnel: [w67 w70] -> w37
      frame False {
      }
      frame True {
        n176 = call "GMLAN TesterPresent.vi"("Parameter"=TesterPresent_Parameter."EntireNetwork", "diag ref in"=w73) -> ("error out"=w71:errorcluster)  [unwired: 7 in, 2 out]
        n177 = Merge Errors(w72, w71) -> (w70:errorcluster)
      }
    }
    n178 = feedback-in #1(w43) -> ()
    n179 = call "Global Stop Actions.vi"("Command"=Stop_Global_Commands."Read", "error in (no error)"=w37, "Stop on Error?"=FALSE, "vi reference"=w31) -> ("error out"=w36:errorcluster, "Latched Stop"=w35:bool)  [unwired: 5 in, 1 out]
    n180 = call "Report Error to Process.vi"("Error"=w36, "This VI"=w34) -> ()  [unwired: 10 in]
  }
  "error out" <- w9
